vi "SYST_CHAN_HOLD.vi"(0 "VISA IN":refnum<visa-resource-name>, 5 "error in":errorcluster) -> (14 "VISA Out":refnum<visa-resource-name>, 19 "error out":errorcluster)   [LabVIEW 2018, in "PNA-X.lvlib"]
doc: "SYSTem:CHANnels:HOLD \n1868\n\n(Write-only) Places all channels in hold mode. To place a single channel in hold mode, use \nSENS:SWE:MODE. \nExamples SYST:CHAN:HOLD \nQuery Syntax Not Applicable \nDefault Not Applicable"
uses:
  PNA-X.lvlib
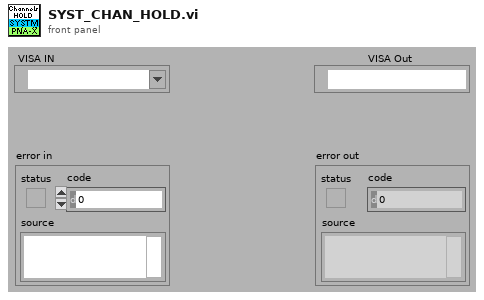
[diagram p1: front panel]
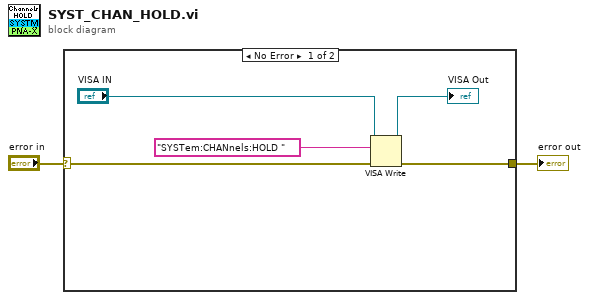
[diagram p0: block diagram]
diagram:
  n1 = case shown="No Error" "error in" {
    selector: "error in" -> [w3 w8]
    tunnel: [w6 w8] -> w1
    frame No Error {
      n2 = VISA Write(VISA resource name="VISA IN", write buffer="SYSTem:CHANnels:HOLD " ("Cmdline"), error in (no error)=w3) -> (VISA resource name out=→"VISA Out":refnum<visa-resource-name>, error out=w6:errorcluster)  [unwired: 1 out]
    }
    frame Error {
    }
  }
  "error out" <- w1
